vi "VFD Initilize.vi"(7 "Slave ID (255)":u8, 8 "error In":errorcluster, 11 "IP Address":string="localhost") -> (0 "error out":errorcluster)   [LabVIEW 2026, in "VFD Library.lvlib"]
uses:
  VFD Library.lvlib
  Private/State Selection FGV.ctl
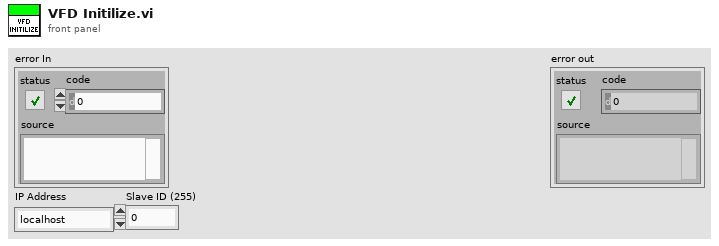
[diagram p1: front panel]
types:
  T1 = typedef "State Selection FGV.ctl" = enum16{"Initilize", "Write Reg", "Write Multiple Reg", "Read Reg", "Write Coil", "Read Coil", "Reset", "Close"}
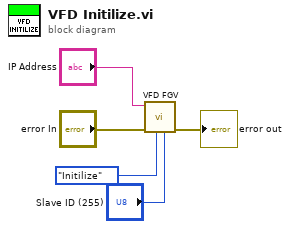
[diagram p0: block diagram]
diagram:
  n1 = call "VFD FGV.vi"("Slave ID (255)"="Slave ID (255)", "State"=State_Selection_FGV."Initilize", "error In"="error In", "IP Address"="IP Address") -> ("error out"=→"error out":errorcluster)  [unwired: 5 in, 2 out]
